vi "LKIF2_StopMeasure.vi"(8 "error in (no error)":errorcluster) -> (0 "error out":errorcluster)   [LabVIEW 2014, in "Keyence LK-G5000.lvlib"]
uses:
  Keyence LK-G5000.lvlib
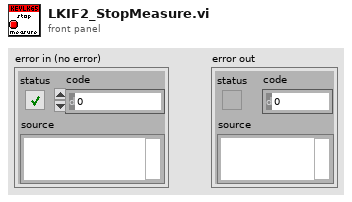
[diagram p1: front panel]
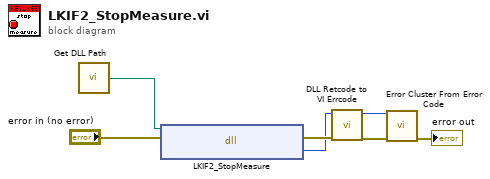
[diagram p0: block diagram]
diagram:
  n1 = call "Get DLL Path.vi"() -> ("DLL Path"=w5:path)  [unwired: 1 in]
  n2 = dll-call lib="C:/Program Files (x86)/National Instruments/LabVIEW 2013/instr.lib/Keyence LK-G5000/LKIF2.dll" fn="LKIF2_StopMeasure"(path in=w5, error in="error in (no error)") -> (error out=w3:errorcluster, "RC"=w2:i32)  [unwired: 1 in, 1 out]
  n3 = call "DLL Retcode to VI Errcode.vi"("error in (no error)"=w3, "DLL Retcode"=w2) -> ("error out"=w6:errorcluster, "VI Errcode"=w7:i32)  [unwired: 8 in]
  n4 = call <vilib>:"Error Cluster From Error Code.vi"("error in (no error)"=w6, "error code (0)"=w7) -> ("error out"=→"error out":errorcluster)  [unwired: 7 in]
